vi "From Variant.vi"(8 "Error In":errorcluster, 10 "Variant":variant, 11 "TD Flt A In":refnum<class "1D Flt.lvclass">) -> (0 "Error Out":errorcluster, 3 "TD Flt A Out":refnum<class "1D Flt.lvclass">)   [LabVIEW 2020, in "NI_VIAnCFGDataStructure.lvlib" / "1D Flt.lvclass"]
doc: "Dynamic dispatch interface for conversion of variant LV data to Tree Data classes."
uses:
  <vilib>/addons/analyzer/VIAnCFGDataStructure/Data Types/Flt Array/1D Flt.lvclass
  <vilib>/addons/analyzer/VIAnCFGDataStructure/Data Types/Flt Array/1D Flt.lvclass/1D Flt.ctl
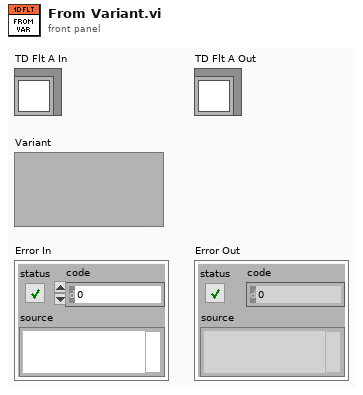
[diagram p1: front panel]
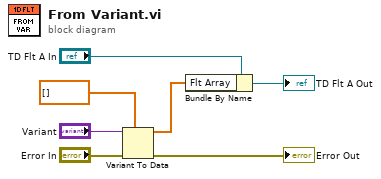
[diagram p0: block diagram]
diagram:
  n1 = Variant To Data(error in="Error In", type=dbl[] [] ("Flt Array"), Variant="Variant") -> (data=w1:dbl[], error out=→"Error Out":errorcluster)
  n2 = Bundle By Name(cluster="TD Flt A In", "Flt Array"=w1) -> (→"TD Flt A Out":refnum<class "1D Flt.lvclass">)
